vi "aoc-2025-d02-1.vi"() -> ()   [LabVIEW 2020]
panel:
  out "sum":u64
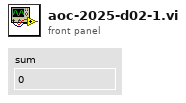
[diagram p1: front panel]
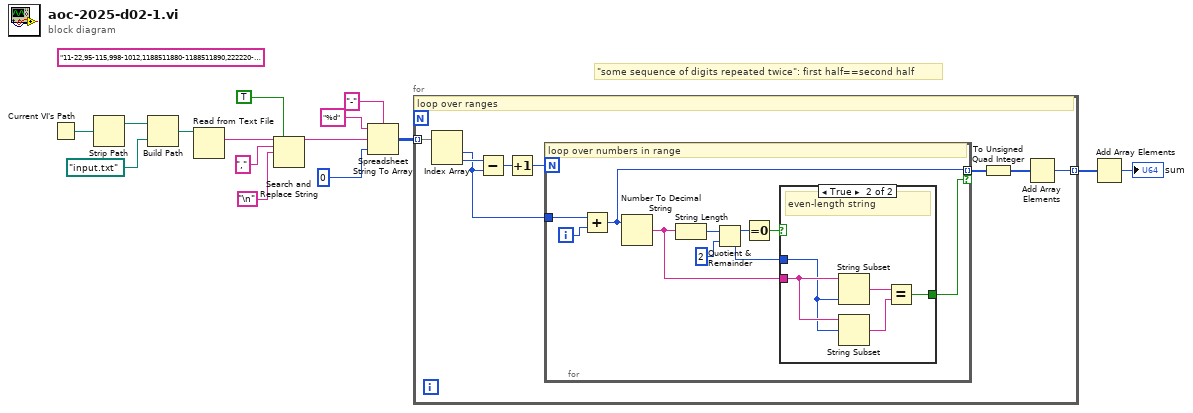
[diagram p0: block diagram]
diagram:
  (unwired) "11-22,95-115,998-1012,1188511880-1188511890,222220-222224,1698522-1698528,446443-446449,38593856-38593862,565653-565659,824824821-824824827,2121212118-2121212124" ("input string")
  # "\"some sequence of digits repeated twice\": first half==second half"
  n1 = Current VI's Path() -> (path=w5:path)
  n2 = Strip Path(path=w5) -> (stripped path=w4:path)  [unwired: 1 out]
  n3 = Build Path(base path=w4, name or relative path=path "input.txt") -> (appended path=w2:path)
  n4 = Read from Text File(file (use dialog)=w2) -> (text=w1:string)  [unwired: 3 in, 3 out]
  n5 = Search and Replace String(replace all?=TRUE ("replace all? (F)"), input string=w1, search string=",", replace string="\n") -> (result string=w9:string)  [unwired: 4 in, 3 out]
  n6 = Spreadsheet String To Array(delimiter (Tab)="-", format string="%d", spreadsheet string=w9, array type (2D Dbl)=u64 0) -> (array=w8:u64[][])
  n7 = for {
    tunnel: w8 -> [w23] mode=indexing
    tunnel: [w17] -> w7 mode=indexing
    # "loop over ranges"
    n8 = Index Array(array=w23) -> (element #1=w20:u64, element #2=w22:u64)  [unwired: 2 in]
    n9 = Subtract(x=w22, y=w20) -> (x-y=w21:u64)
    n10 = Increment(x=w21) -> (x+1=w19:u64)
    n11 = for {
      N: w19 -> [_]
      tunnel: w20 -> [w33]
      tunnel: [w25] -> w18 mode=indexing if=w24
      i -> [w32]
      # "loop over numbers in range"
      n12 = Add(x=w33, y=w32) -> (x+y=w25:u64)
      n13 = Number To Decimal String(number=w25) -> (decimal integer string=w29:string)  [unwired: 1 in]
      n14 = String Length(string=w29) -> (length=w28:i32)
      n15 = Quotient & Remainder(x=w28, y=2) -> (x-y*floor(x/y)=w31:i32, floor(x/y)=w27:i32)
      n16 = Equal To 0?(x=w31) -> (x = 0?=w30:bool)
      n17 = case shown="True" w30 {
        tunnel: w29 -> [_ w38]
        tunnel: w27 -> [_ w34]
        tunnel: [_ w35] -> w24
        frame False {
        }
        frame True {
          # "even-length string"
          n18 = String Subset(string=w38, length (rest)=w34) -> (substring=w37:string)  [unwired: 1 in]
          n19 = String Subset(string=w38, offset (0)=w34) -> (substring=w36:string)  [unwired: 1 in]
          n20 = Equal?(x=w37, y=w36) -> (x = y?=w35:bool)
        }
      }
    }
    n21 = To Unsigned Quad Integer(1:w18) -> (0:w16:u64[])
    n22 = Add Array Elements(numeric array=w16) -> (sum=w17:u64)
  }
  n23 = Add Array Elements(numeric array=w7) -> (sum=→"sum":u64)
